vi "Get Measurement_v1_GetMetadataResponse.vi"(8 "error in (no error)":errorcluster, 11 "gRPCid":T7) -> (0 "error out":errorcluster, 2 "Message Data":T1, 3 "gRPCid out":T7)   [LabVIEW 2020, in "LineRegulation.lvlib" / "MeasurementService_Template.lvclass"]
uses:
  MeasurementService_Template.lvclass
  <vilib>/gRPC/LabVIEW gRPC Library/Server API/typeDefs/grpcId.ctl
  Measurement_v1_GetMetadataResponse_Data.ctl
  Measurement_v1_MeasurementDetails/Measurement_v1_MeasurementDetails_Data.ctl
  Measurement_v1_MeasurementParameters/Measurement_v1_MeasurementParameters_Data.ctl
  Measurement_v1_ConfigurationParameter/Measurement_v1_ConfigurationParameter_Data.ctl
  Measurement_v1_OutputParameter/Measurement_v1_OutputParameter_Data.ctl
  Measurement_v1_UserInterfaceDetails/Measurement_v1_UserInterfaceDetails_Data.ctl
  a51dd2a7-b5c1-4c09-9df4-8cd9d3bd0c19.vi
  <vilib>/gRPC/LabVIEW gRPC Library/Server API/Server/Get Server DLL Path.vi
  <vilib>/gRPC/LabVIEW gRPC Library/gprc-lvsupport-release.lvlib
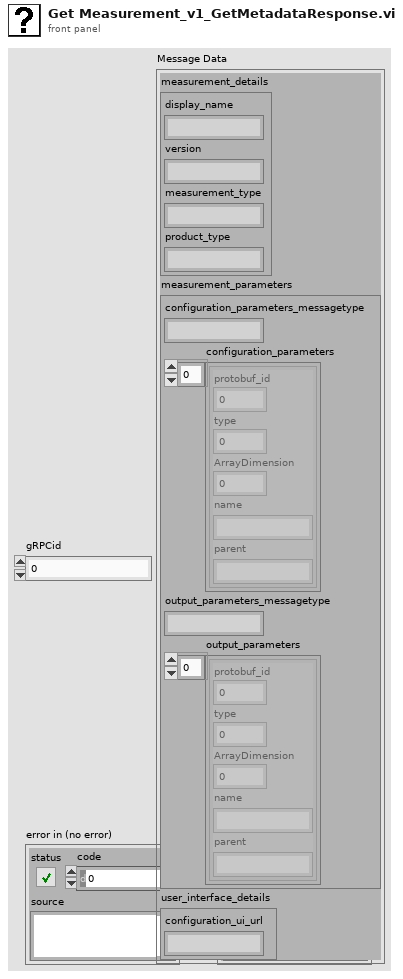
[diagram p1: front panel]
types:
  T1 = typedef "LineRegulation.lvlib/MeasurementService_Template.lvclass/Measurement_v1_GetMetadataResponse_Data.ctl" = cluster{"measurement_details":T2, "measurement_parameters":T3, "user_interface_details":T6}
  T2 = typedef "LineRegulation.lvlib/MeasurementService_Template.lvclass/Measurement_v1_MeasurementDetails_Data.ctl" = cluster{"display_name":string, "version":string, "measurement_type":string, "product_type":string}
  T3 = typedef "LineRegulation.lvlib/MeasurementService_Template.lvclass/Measurement_v1_MeasurementParameters_Data.ctl" = cluster{"configuration_parameters_messagetype":string, "configuration_parameters":T4[], "output_parameters_messagetype":string, "output_parameters":T5[]}
  T4 = typedef "LineRegulation.lvlib/MeasurementService_Template.lvclass/Measurement_v1_ConfigurationParameter_Data.ctl" = cluster{"protobuf_id":i32, "type":i32, "ArrayDimension":i32, "name":string, "parent":string}
  T5 = typedef "LineRegulation.lvlib/MeasurementService_Template.lvclass/Measurement_v1_OutputParameter_Data.ctl" = cluster{"protobuf_id":i32, "type":i32, "ArrayDimension":i32, "name":string, "parent":string}
  T6 = typedef "LineRegulation.lvlib/MeasurementService_Template.lvclass/Measurement_v1_UserInterfaceDetails_Data.ctl" = cluster{"configuration_ui_url":string}
  T7 = typedef "gprc-lvsupport-release.lvlib/grpcId.ctl" = u64
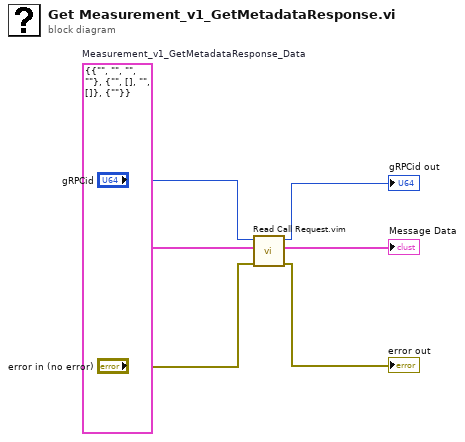
[diagram p0: block diagram]
diagram:
  w2 = T1 {"measurement_details"={"display_name"="", "version"="", "measurement_type"="", "product_type"=""}, "measurement_parameters"={"configuration_parameters_messagetype"="", "configuration_parameters"=[], "output_parameters_messagetype"="", "output_parameters"=[]}, "user_interface_details"={"configuration_ui_url"=""}}  # Measurement_v1_GetMetadataResponse_Data
  n1 = call "Read Call Request.vim"("error in (no error)"="error in (no error)", "Data Type"=w2, "gRPCid in"="gRPCid") -> ("error out"=→"error out":errorcluster, "Request Data"=→"Message Data":T1, "gRPCid out"=→"gRPCid out":T7)  [unwired: 6 in]
